vi "getData.vi"(8 "error in (no error)":errorcluster, 11 "Context In":refnum<class "Context.lvclass"> caption="Context DVR In") -> (0 "error out":errorcluster, 2 "ContextData.lvclass":refnum<class "ContextData.lvclass">, 3 "Context Out":refnum<class "Context.lvclass"> caption="Context DVR In")   [LabVIEW 2020, in "Context.lvclass"]
uses:
  Context.lvclass
  ContextData/ContextData.lvclass
  Context.lvclass/Context.ctl
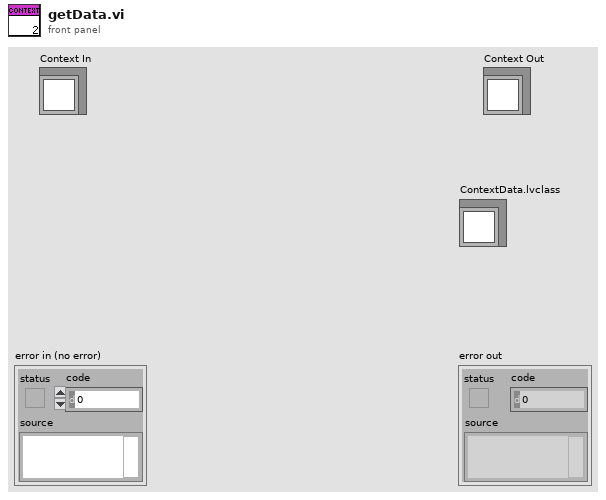
[diagram p1: front panel]
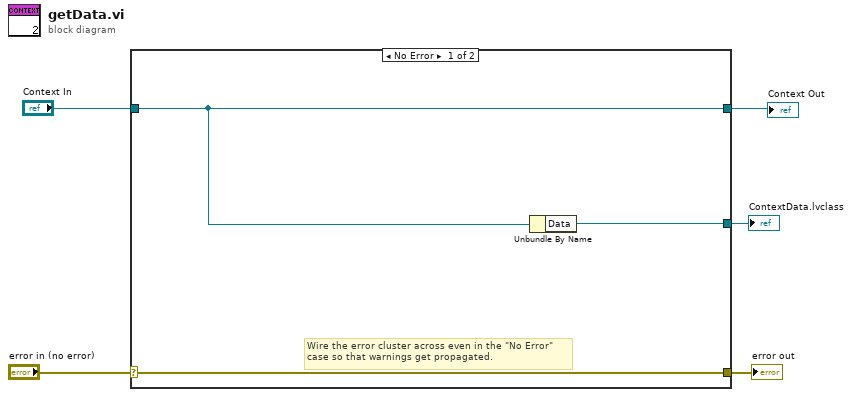
[diagram p0: block diagram]
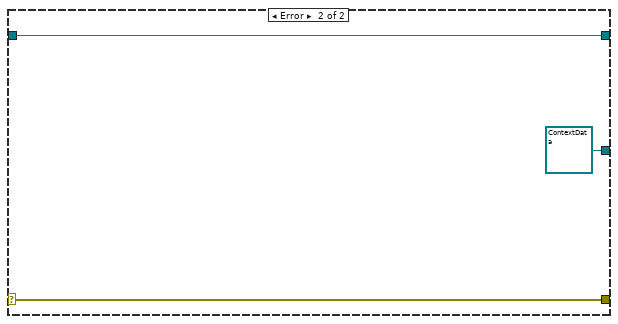
[diagram p2: hidden frame]
diagram:
  n1 = case shown="No Error" "error in (no error)" {
    selector: "error in (no error)" -> [w8 w11]
    tunnel: [w8 w11] -> w4
    tunnel: [w6 w10] -> w1
    tunnel: "Context In" -> [w6 w10]
    tunnel: [w7 refnum<class "ContextData.lvclass"> refnum ("Data")] -> w3
    frame No Error {
      # "Wire the error cluster across even in the \"No Error\"\ncase so that warnings get propagated."
      n2 = Unbundle By Name(w6) -> ("Data"=w7:refnum<class "ContextData.lvclass">)
    }
    frame Error {
    }
  }
  "error out" <- w4
  "ContextData.lvclass" <- w3
  "Context Out" <- w1
